vi "Set File Property.vi"(5 "Value":variant, 7 "Name":string, 8 "error in (no error)":errorcluster, 11 "TDMS Log File Specification in":refnum<class "TDMS Log File Specification.lvclass">) -> (0 "error out":errorcluster, 3 "TDMS Log File Specification out":refnum<class "TDMS Log File Specification.lvclass">)   [LabVIEW 2015, in "Waveform Data Logger Shared.lvlib" / "TDMS Log File Specification.lvclass"]
uses:
  TDMS Log File Specification.lvclass
  TDMS Log File Specification.lvclass/TDMS Log File Specification.ctl
  Property Specification.ctl
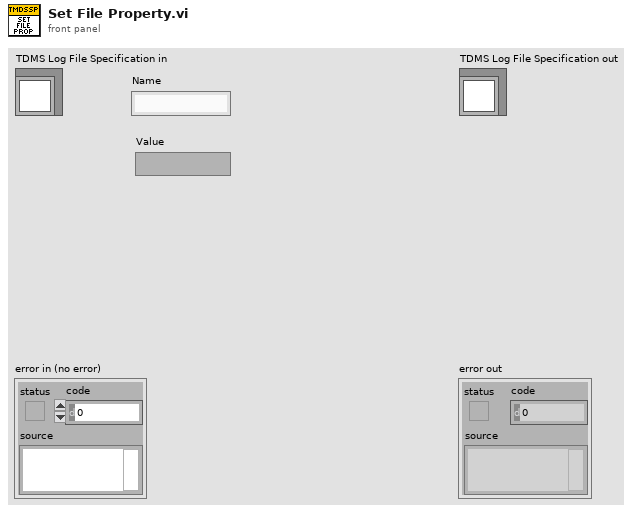
[diagram p1: front panel]
types:
  T1 = typedef "Waveform Data Logger Shared.lvlib/TDMS Log File Specification.lvclass/Property Specification.ctl" = cluster{"Name":string, "Value":variant}
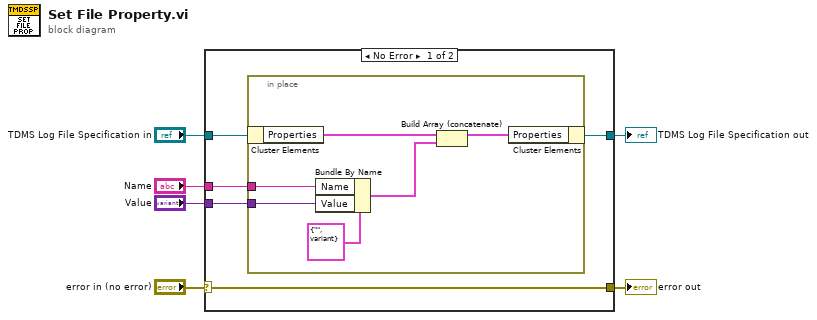
[diagram p0: block diagram]
diagram:
  n1 = case shown="No Error" "error in (no error)" {
    selector: "error in (no error)" -> [w11 w19]
    tunnel: [w11 w19] -> w5
    tunnel: [w7 w18] -> w3
    tunnel: "TDMS Log File Specification in" -> [w10 w18]
    tunnel: "Name" -> [w9 _]
    tunnel: "Value" -> [w8 _]
    frame No Error {
      n2 = in-place {
        in-place-border: w9 -> [w15]
        in-place-border: w8 -> [w14]
        n3 = in-place-cluster #1(w10) -> ("Properties"=w17:T1[])
        n4 = Bundle By Name(cluster=T1 {"Name"="", "Value"=variant} ("Property"), "Name"=w15, "Value"=w14) -> (w13:T1)
        n5 = Build Array (concatenate)(w17, w13) -> (w12:T1[])
        n6 = in-place-cluster #1("Properties"=w12) -> (w7:refnum<class "TDMS Log File Specification.lvclass">)
      }
    }
    frame Error {
    }
  }
  "error out" <- w5
  "TDMS Log File Specification out" <- w3
